vi "Convert Table to Form.vi"(8 "error in (no error)":errorcluster, 10 "Table Object":refnum<class "Basic Table.lvclass">, 11 "Basic Form in":refnum<class "Basic Form.lvclass">) -> (0 "error out":errorcluster, 3 "Basic Form out":refnum<class "Basic Form.lvclass">)   [LabVIEW 2020, in "Form.lvlib" / "Basic Form.lvclass"]
uses:
  Basic Form.lvclass
  C:/Users/User/Desktop/Raman Program/Database OOP/source/Database OOP/Table Libraries/Basic Table/Basic Table Class/Basic Table.lvclass
  Basic Table/Basic Table Class/Basic Table.lvclass
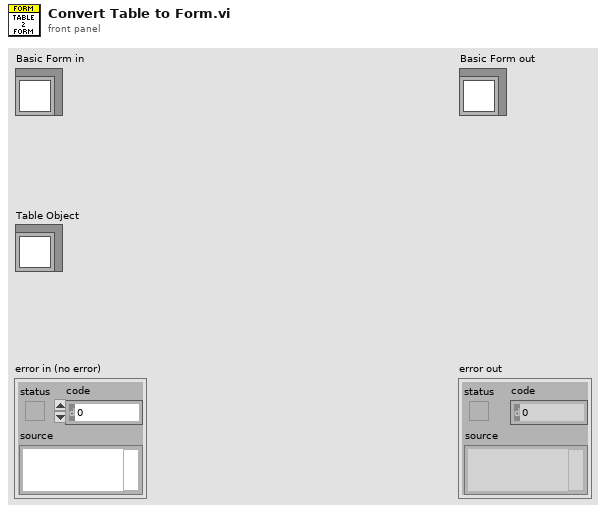
[diagram p1: front panel]
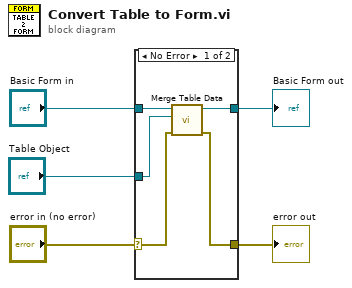
[diagram p0: block diagram]
diagram:
  n1 = case shown="No Error" "error in (no error)" {
    selector: "error in (no error)" -> [w7 w12]
    tunnel: [w6 w12] -> w4
    tunnel: [w8 w11] -> w2
    tunnel: "Basic Form in" -> [w9 w11]
    tunnel: "Table Object" -> [w10 _]
    frame No Error {
      n2 = call "Merge Table Data.vi"("error in (no error)"=w7, "Table to Merge"=w10, "Basic Table in"=w9) -> ("error out"=w6:errorcluster, "Basic Table out"=w8:refnum<class "Basic Form.lvclass">)  [unwired: 7 in]
    }
    frame Error {
    }
  }
  "error out" <- w4
  "Basic Form out" <- w2
